vi "Mode Page.vi"(8 "Error In":errorcluster, 11 "Sample Test Template in":refnum<class "Sample Test Template.lvclass">) -> (0 "Error Out":errorcluster, 3 "Sample Test Template out":refnum<class "Sample Test Template.lvclass">)   [LabVIEW 2020, in "Sample Test Template.lvclass"]
doc: "Mode page Template"
uses:
  Sample Test Template.lvclass
  Parent/Typedef/User Event Controls.ctl
  Parent/Typedef/Queue Driver Controls.ctl
  Parent/Test.lvclass
panel:
  # "Sample Mode Page"
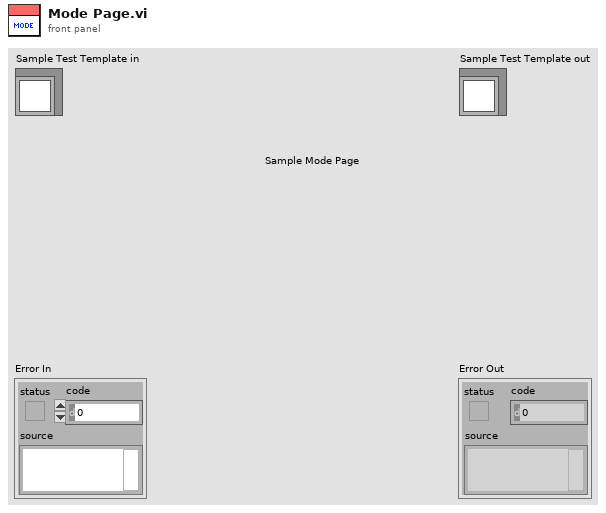
[diagram p1: front panel]
types:
  T1 = typedef "Test.lvclass/Queue Driver Controls.ctl" = enum16{"Create Queue", "Enqueue", "Dequeue", "Enstack", "Flush Queue", "Release Queue"}
  T2 = typedef "Test.lvclass/User Event Controls.ctl" = enum16{"Create", "Generate", "Run Test", "Get Ref", "Destroy"}
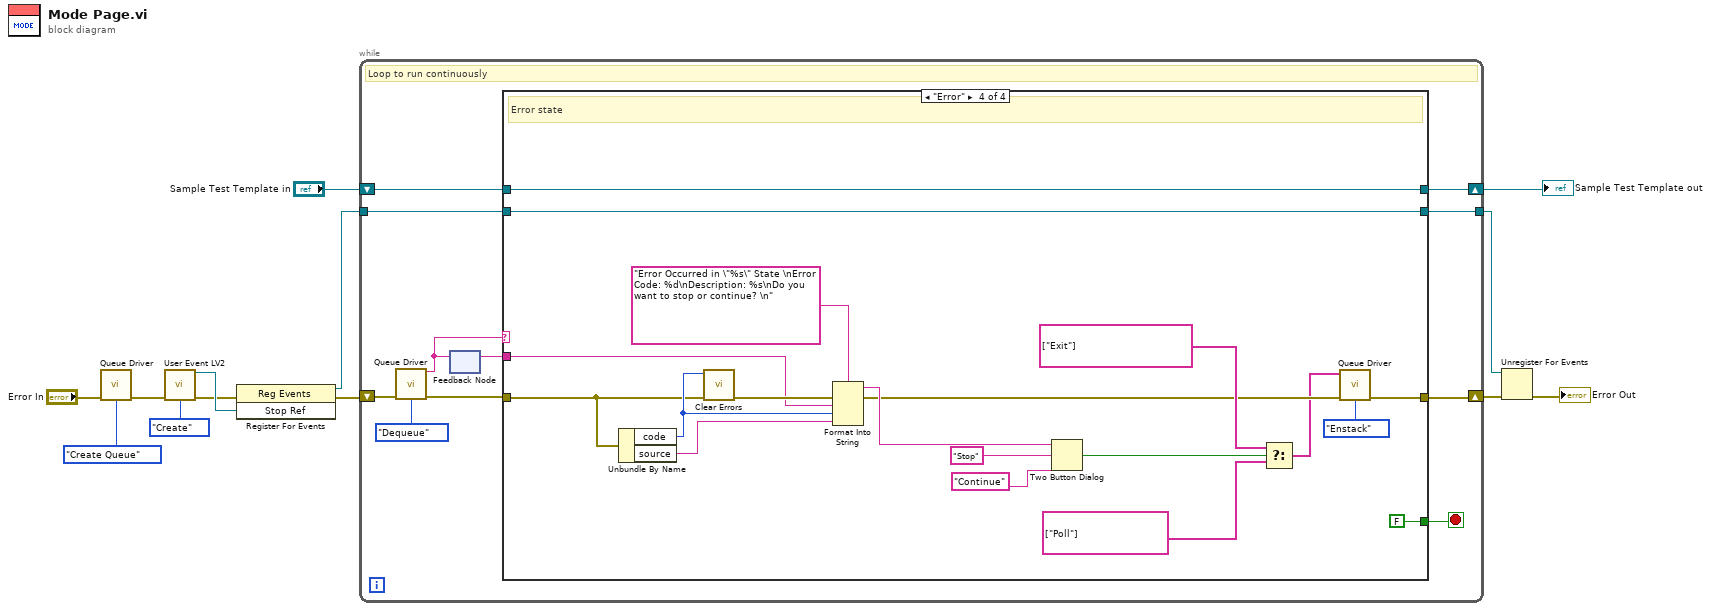
[diagram p0: block diagram]
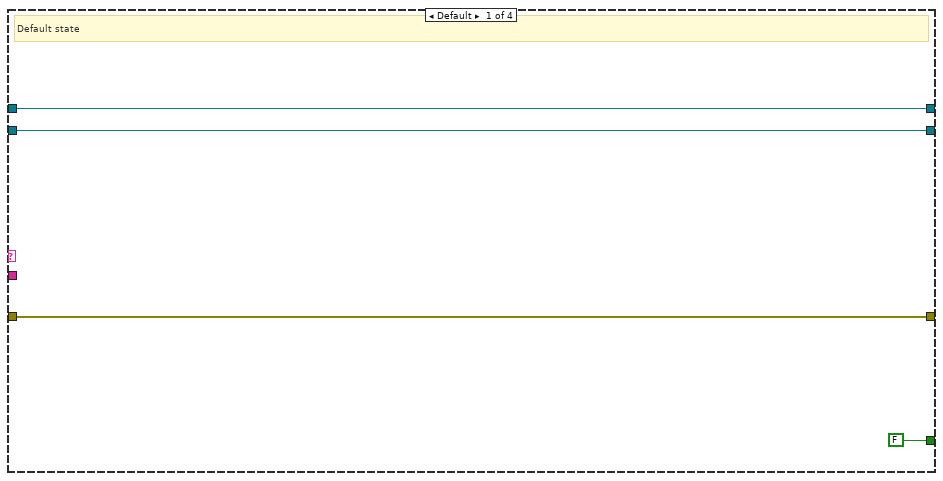
[diagram p2: hidden frame]
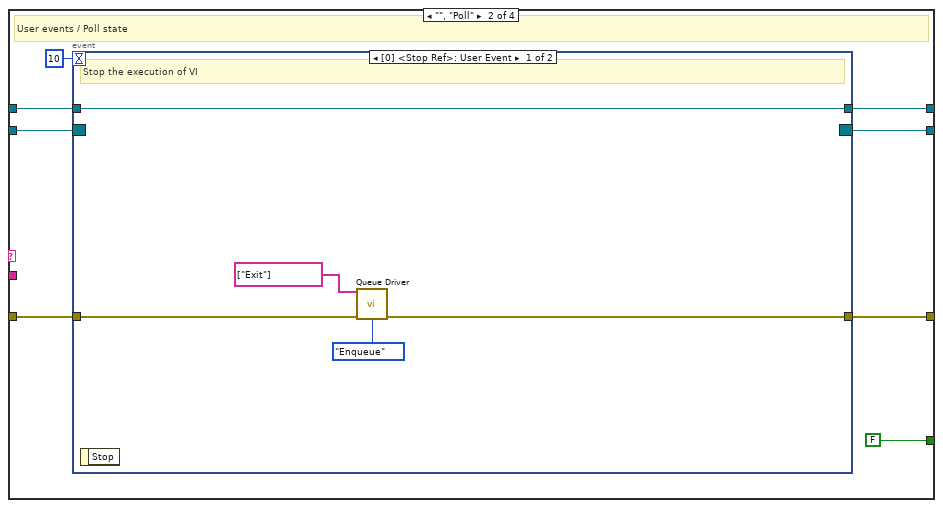
[diagram p3: hidden frame]
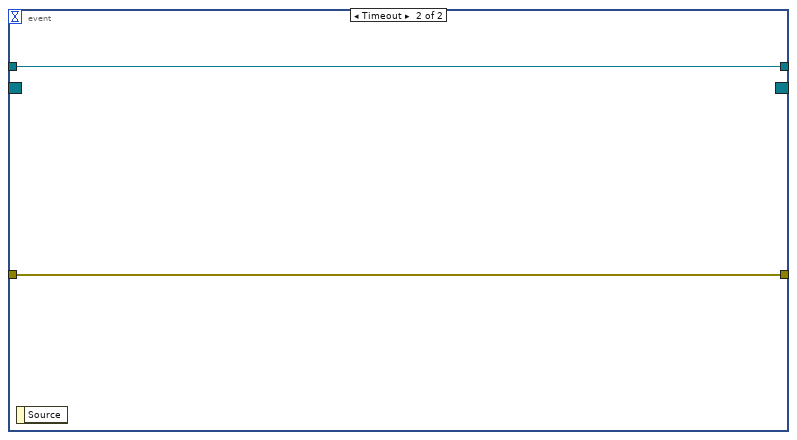
[diagram p4: hidden frame]
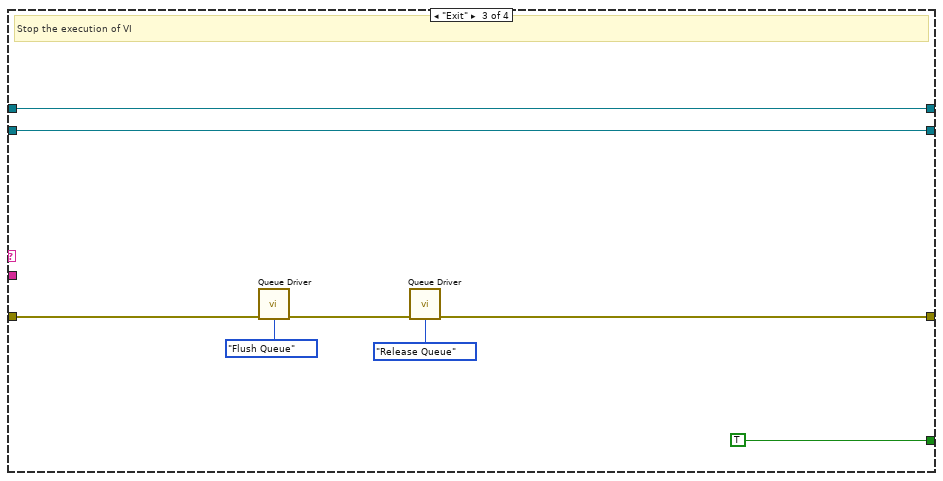
[diagram p5: hidden frame]
diagram:
  n1 = call "Queue Driver.vi"("Error in"="Error In", "Queue Controls"=Queue_Driver_Controls."Create Queue") -> ("Error out"=w2:errorcluster)  [unwired: 12 in, 1 out]
  n2 = call "User Event LV2.vi"("Error In"=w2, "User event controls"=User_Event_Controls."Create") -> ("Stop Ref"=w6:refnum<user-event>, "Error Out"=w5:errorcluster)  [unwired: 11 in, 1 out]
  n3 = register-events(error in=w5, w6) -> (reference out=w13:refnum<event-registration>, error out=w12:errorcluster)  [unwired: 1 in]
  n4 = while {
    tunnel: w13 -> [w24]
    shift-right: [w22] -> w8
    shift-left: "Sample Test Template in" -> [w23]
    shift-right: [w21] -> w11
    shift-left: w12 -> [w17]
    tunnel: [w20] -> w10
    stop <- w19 stop-if-true
    # "Loop to run continuously"
    n5 = call "Queue Driver.vi"("Error in"=w17, "Queue Controls"=Queue_Driver_Controls."Dequeue") -> ("Dequeue Element"=w16:string, "Error out"=w15:errorcluster)  [unwired: 12 in]
    n6 = feedback-in #1(w16) -> ()
    n7 = feedback #1() -> (w18:string)  [unwired: 1 in]
    n8 = case shown="\"Error\"" w16 {
      tunnel: w24 -> [w26 w36 w50 w58]
      tunnel: w15 -> [w27 w35 w48 w60]
      tunnel: w23 -> [w28 w34 w51 w57]
      tunnel: [w28 w33 w51 w57] -> w22
      tunnel: [w27 w30 w46 w53] -> w21
      tunnel: [w26 w32 w50 w58] -> w20
      tunnel: [FALSE FALSE TRUE FALSE ("ADC_")] -> w19
      tunnel: w18 -> [_ _ _ w59]
      frame Default {
        # "Default state"
      }
      frame "", "Poll" {
        # "User events / Poll state"
        n9 = event shown="[0] <Stop Ref>: User Event" {
          selector: w36 -> [_ _]
          dyn-events: [_ _] -> w32
          timeout: 10 -> [_ _]
          tunnel: w35 -> [w40 w42]
          tunnel: w34 -> [w41 w43]
          tunnel: [w41 w43] -> w33
          tunnel: [w39 w42] -> w30
          event User Event {
            # "Stop the execution of VI"
            n10 = event-data() -> ()  [unwired: 1 in, 1 out]
            n11 = call "Queue Driver.vi"("States"=string[] ["Exit"], "Error in"=w40, "Queue Controls"=Queue_Driver_Controls."Enqueue") -> ("Error out"=w39:errorcluster)  [unwired: 11 in, 1 out]
          }
          event Timeout {
            n12 = event-data() -> ()  [unwired: 1 in, 1 out]
          }
        }
      }
      frame "Exit" {
        # "Stop the execution of VI"
        n13 = call "Queue Driver.vi"("Error in"=w48, "Queue Controls"=Queue_Driver_Controls."Flush Queue") -> ("Error out"=w47:errorcluster)  [unwired: 12 in, 1 out]
        n14 = call "Queue Driver.vi"("Error in"=w47, "Queue Controls"=Queue_Driver_Controls."Release Queue") -> ("Error out"=w46:errorcluster)  [unwired: 12 in, 1 out]
      }
      frame "Error" {
        # "Error state"
        n15 = Unbundle By Name(w60) -> ("code"=w68:i32, "source"=w67:string)
        n16 = call <vilib>:"Clear Errors.vi"("error in (no error)"=w60, "specific error code to clear (0: all)"=w68) -> ("error out"=w70:errorcluster)  [unwired: 4 in, 1 out]
        n17 = Format Into String(format string="Error Occurred in \"%s\" State \nError Code: %d\nDescription: %s\nDo you want to stop or continue? \n", error in=w70, w59, w68, w67) -> (resulting string=w66:string, error out=w55:errorcluster)  [unwired: 1 in]
        n18 = Two Button Dialog(message=w66, 1:"Continue" ("F button name (\"Cancel\")"), 2:"Stop" ("T button name (\"OK\")")) -> (T button?=w63:bool)
        n19 = Select(t=string[] ["Exit"] ("States"), s=w63, f=string[] ["Poll"] ("States")) -> (s? t:f=w54:string[])
        n20 = call "Queue Driver.vi"("States"=w54, "Error in"=w55, "Queue Controls"=Queue_Driver_Controls."Enstack") -> ("Error out"=w53:errorcluster)  [unwired: 11 in, 1 out]
      }
    }
  }
  "Sample Test Template out" <- w8
  n21 = Unregister For Events(event registration refnum=w10, error in=w11) -> (error out=→"Error Out":errorcluster)
